vi "Analog Bank Read.vi"(8 "error in (no error)":errorcluster, 11 "TCP Network Connection in":refnum<k5>) -> (0 "error out":errorcluster, 2 "Measurements":sgl[](array[numeric]), 3 "TCP Network Connection out":refnum<k5>)   [LabVIEW 2024, in "OptoMMP.lvlib"]
doc: "Performs an analog bank read on the specified TCP network and returns an array of 64 float values. NaN is written to channels if a communication error occurs.\n\nIn order from top to bottom, the \"Measurements\" array corresponds to channel 0 of module 0 through channel 4 of module 15 (increasing order). \"Analog Bank Read\" must be preceded by \"OptoMMP Open Connection\" or \"Powerup Clear\" if a new connection has been established.\n\nLast updated: 8/6/2025"
uses:
  <instrlib>/OptoMMP/OptoMMP.lvlib
panel:
  # "Copyright (c) 2025 California Institute of Technology (Caltech).\nU.S. Government sponsorship acknowledged.\n\nLicensed under the Apache License, Version 2.0 (the \"License\");\nyou may not use this file except in compliance with the License.\nYou may obtain a copy of the License at\n\n    http://www.apache.org/licenses/LICENSE-2.0\n\nUnless required by applicable law or agreed to in writing, software\ndistributed under the License is distributed on an \"AS IS\" BASIS,\nWITHOUT WARRANTIES OR CONDITIONS OF ANY KIND, either express or implied.\nSee the License for the specific language governing permissions and\nlimitations under the License."
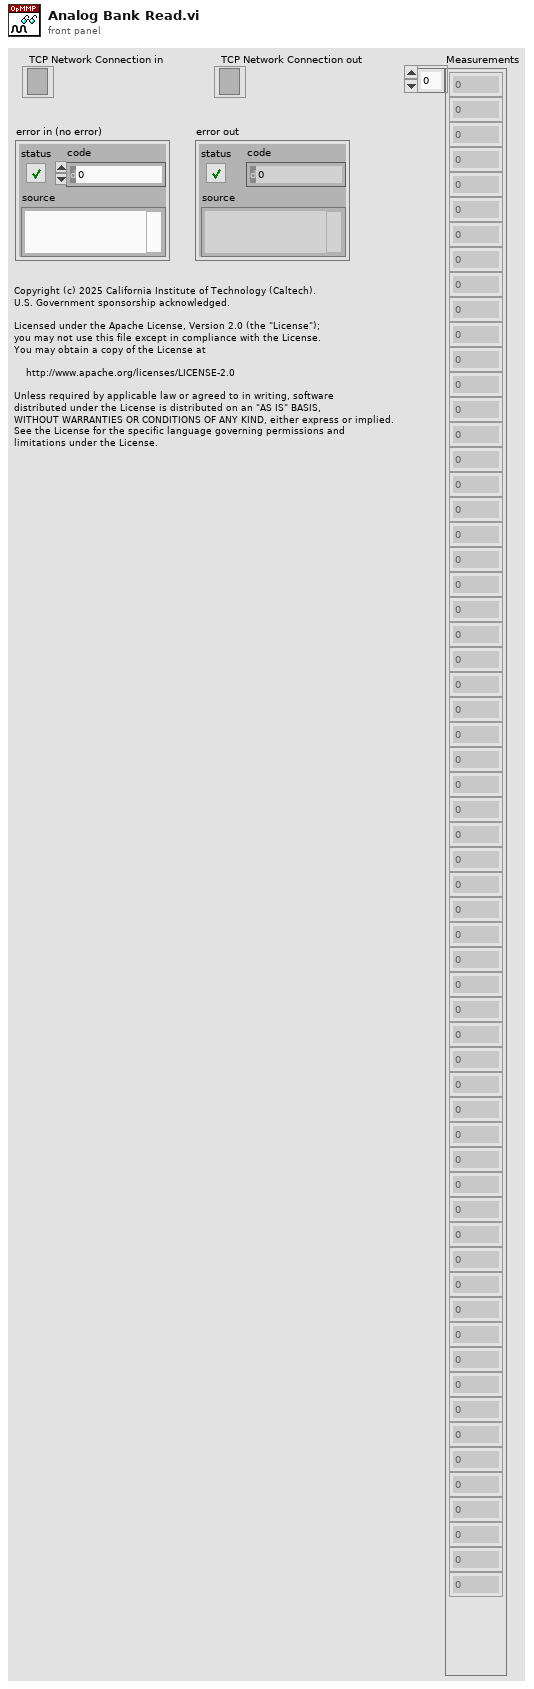
[diagram p1: front panel]
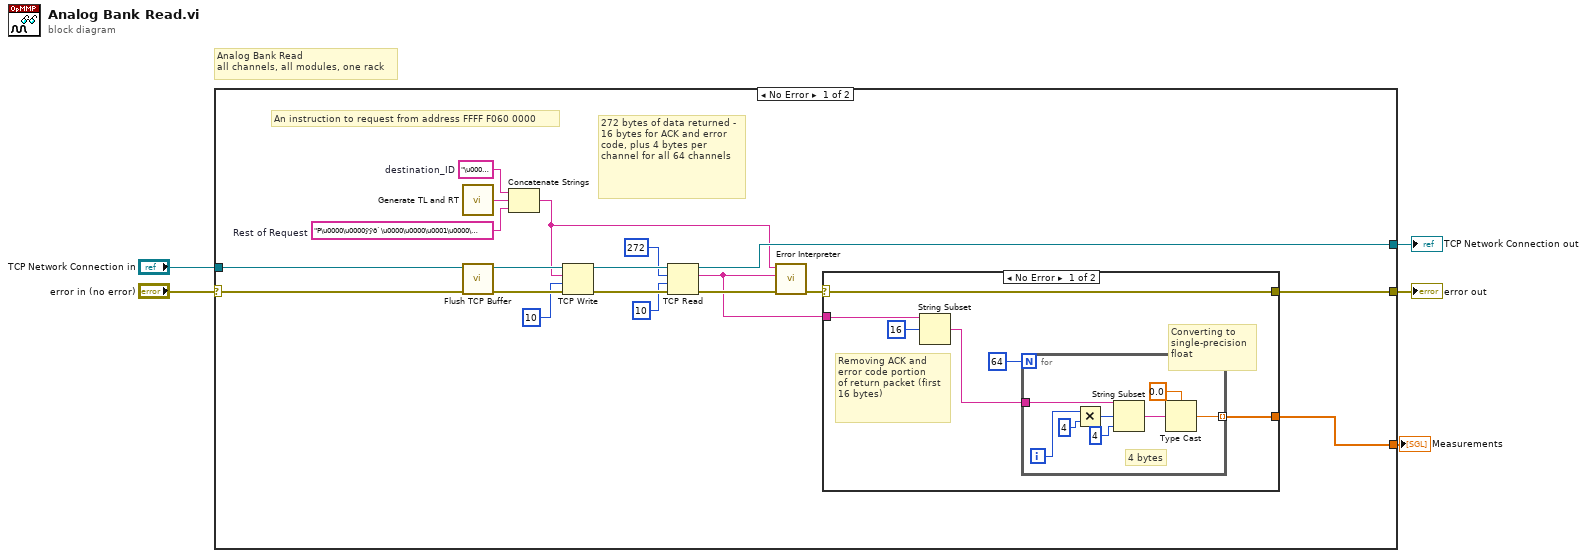
[diagram p0: block diagram]
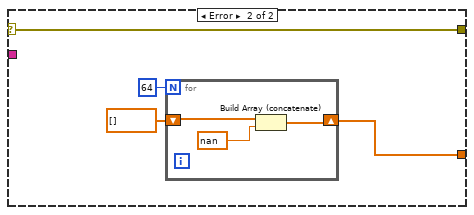
[diagram p2: hidden frame]
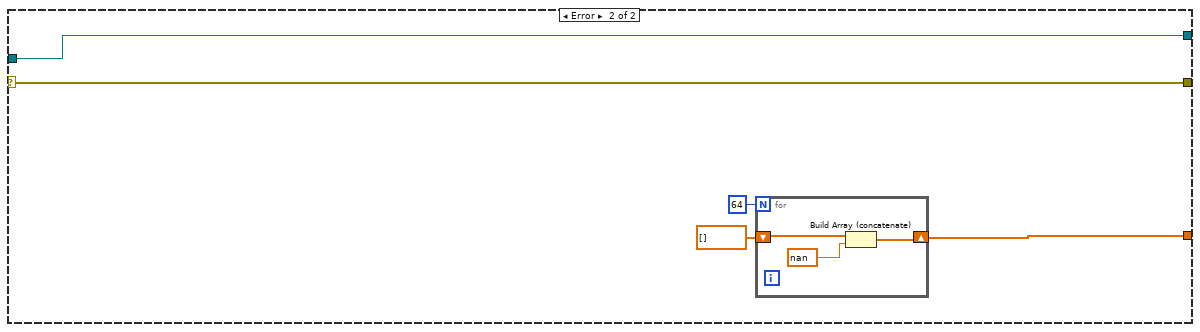
[diagram p3: hidden frame]
diagram:
  # "Analog Bank Read\nall channels, all modules, one rack"
  n1 = case shown="No Error" "error in (no error)" {
    selector: "error in (no error)" -> [w13 w47]
    tunnel: [w6 w47] -> w5
    tunnel: [w24 w46] -> w4
    tunnel: "TCP Network Connection in" -> [w23 w46]
    tunnel: [w22 w48] -> w2
    frame No Error {
      w9 = "P\u0000\u0000ÿÿð`\u0000\u0000\u0001\u0000\u0000\u0000"  # Rest of Request
      w10 = "\u0000\u0000"  # destination_ID
      # "272 bytes of data returned - 16 bytes for ACK and error code, plus 4 bytes per channel for all 64 channels"
      # "An instruction to request from address FFFF F060 0000"
      n2 = call <instrlib>:"Generate TL and RT.vi"() -> ("tl + rt"=w11:string)
      n3 = call <instrlib>:"Flush TCP Buffer.vi"("error in (no error)"=w13, "TCP Network Connection in"=w23) -> ("error out"=w17:errorcluster, "TCP Network Connection out"=w16:refnum<k5>)  [unwired: 8 in]
      n4 = Concatenate Strings(w10, w11, w9) -> (w8:string)
      n5 = TCP Write(connection ID=w16, data in=w8, error in (no error)=w17, 9:10 ("timeout ms (25000)")) -> (connection ID out=w21:refnum<k5>, error out=w20:errorcluster)  [unwired: 1 out]
      n6 = TCP Read(connection ID=w21, bytes to read=272, error in (no error)=w20, 9:10 ("timeout ms (25000)")) -> (connection ID out=w24:refnum<k5>, data out=w14:string, error out=w15:errorcluster)  [unwired: 1 in]
      n7 = call <instrlib>:"Error Interpreter.vi"("request packet"=w8, "response packet"=w14, "error in (no error)"=w15) -> ("error out"=w7:errorcluster)  [unwired: 7 in]
      n8 = case shown="No Error" w7 {
        selector: w7 -> [w25 w39]
        tunnel: [w28 w42] -> w22
        tunnel: w14 -> [w27 _]
        tunnel: [w25 w39] -> w6
        frame No Error {
          # "Removing ACK and \nerror code portion \nof return packet (first\n16 bytes)"
          # "Converting to \nsingle-precision\nfloat"
          n9 = String Subset(string=w27, offset (0)=16) -> (substring=w30:string)  [unwired: 1 in]
          n10 = for {
            N: 64 -> [_]
            tunnel: w30 -> [w38]
            tunnel: [w35] -> w28 mode=indexing
            i -> [w33]
            # "4 bytes"
            n11 = Multiply(x=w33, y=4 ("length (rest)")) -> (x*y=w31:i32)
            n12 = String Subset(string=w38, offset (0)=w31, length (rest)=4 ("length (rest)")) -> (substring=w36:string)
            n13 = Type Cast(type=sgl 0.0, x=w36) -> (*(type *) &x=w35:sgl)
          }
        }
        frame Error {
          n14 = for {
            N: 64 -> [_]
            shift-right: [w44] -> w42
            shift-left: sgl[] [] -> [w43]
            n15 = Build Array (concatenate)(w43, sgl nan) -> (w44:sgl[])
          }
        }
      }
    }
    frame Error {
      n16 = for {
        N: 64 -> [_]
        shift-right: [w52] -> w48
        shift-left: sgl[] [] -> [w51]
        n17 = Build Array (concatenate)(w51, sgl nan) -> (w52:sgl[])
      }
    }
  }
  "TCP Network Connection out" <- w4
  "error out" <- w5
  "Measurements" <- w2
